vi "Cell I Set All.vi"(7 "Box ID":u8, 8 "error in (no error)":errorcluster, 9 "Sink I All":dbl, 10 "Source I All":dbl, 11 "ENET in":refnum<class "ENET_BS120x.lvclass">) -> (0 "error out":errorcluster, 3 "ENET out":refnum<class "ENET_BS120x.lvclass">)   [LabVIEW 2021, in "BS120x Driver.lvlib" / "ENET_BS120x.lvclass"]
uses:
  ENET_BS120x.lvclass
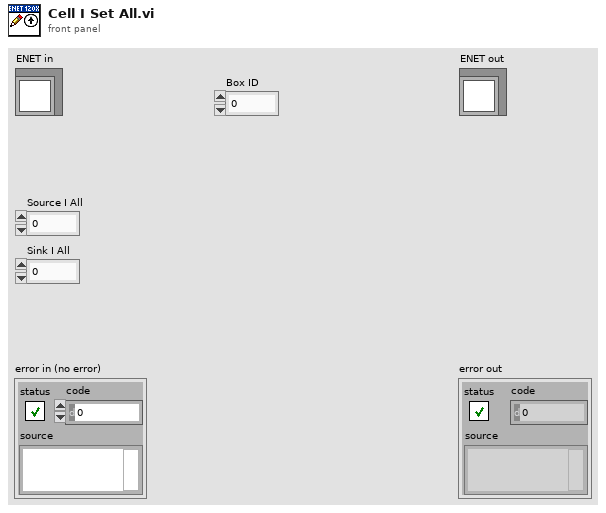
[diagram p1: front panel]
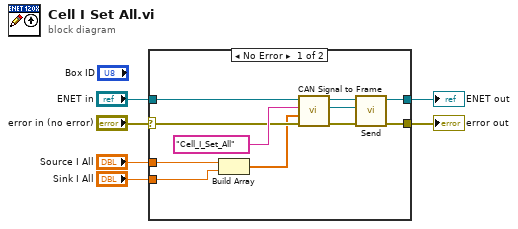
[diagram p0: block diagram]
diagram:
  n1 = case shown="No Error" "error in (no error)" {
    selector: "error in (no error)" -> [w12 w18]
    tunnel: [w13 w18] -> w6
    tunnel: "Source I All" -> [w11 _]
    tunnel: "Sink I All" -> [w10 _]
    tunnel: "ENET in" -> [w9 w19]
    tunnel: [w7 w19] -> w1
    frame No Error {
      n2 = Build Array(w11, w10) -> (w8:dbl[])
      n3 = call "CAN Signal to Frame.vi"("error in (no error)"=w12, "Data Array"=w8, "Frame"="Cell_I_Set_All", "ENET in"=w9) -> ("error out"=w17:errorcluster, "Data"=w16:refnum<class "Data.lvclass">, "ENET out"=w15:refnum<class "ENET_BS120x.lvclass">)  [unwired: 5 in]
      n4 = call "Send.vi"("error in (no error)"=w17, "Data"=w16, "ENET in"=w15) -> ("error out"=w13:errorcluster, "ENET out"=w7:refnum<class "ENET_BS120x.lvclass">)  [unwired: 7 in]
    }
    frame Error {
    }
  }
  "error out" <- w6
  "ENET out" <- w1
